vi "0_Augment_Dataset.vi"() -> ()   [LabVIEW 2020]
uses:
  <vilib>/vision/NI_Vision_Development_Module.lvlib
panel:
  out "File Data Type":i32(ring)=5 items=["1 bit", "2 bits", "4 bits", "8 bits", "12 bits (unsigned)", "16 bits (unsigned)", "16 bits (signed)", "16 bits (RGB chunky)", "24 bits (RGB chunky)", "24 bits (RGB planar)", "32 bits (unsigned)", "32 bits (signed)", "32 bits (RGB chunky)", "32 bits (float)", "48 bits (Complex 2x24 int)", "64 bits (Complex 2x32 float)", "reserved", "24 bits (HSL)", "48 bits (RGB chunky)", "64 bits (RGB chunky)"]
  out "Image Type":T1=7 items=["Grayscale (U8)", "Grayscale (I16)", "Grayscale (SGL)", "Complex (CSG)", "RGB (U32)", "HSL (U32)", "RGB (U64)", "Grayscale (U16)"]
  out "error out":errorcluster
  in  "error in (no error)":errorcluster
  in  "Image Path":path=path "D:/Ngene/Projects_SVN/LV_DNN_Projects/2022/2022_09_14_Andrzej Czechowski_Comex/2_Dataset/2022_10_04_Initial_Dataset/orig_train_test_aug_FR0"
  out "No of Images":i32=756
  out "Progress":i32=755
  # "Description:\nThis VI increases datset size by a facor of 8 by applyig vertical and horizontal flipping and rotation by 90, 180 and 270 degrees."
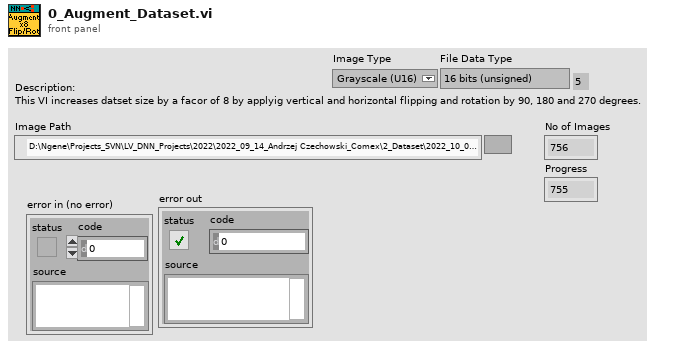
[diagram p1: front panel]
types:
  T1 = typedef "Image Type" = u32
  T2 = typedef "IMAQ Image.ctl" = refnum<image>
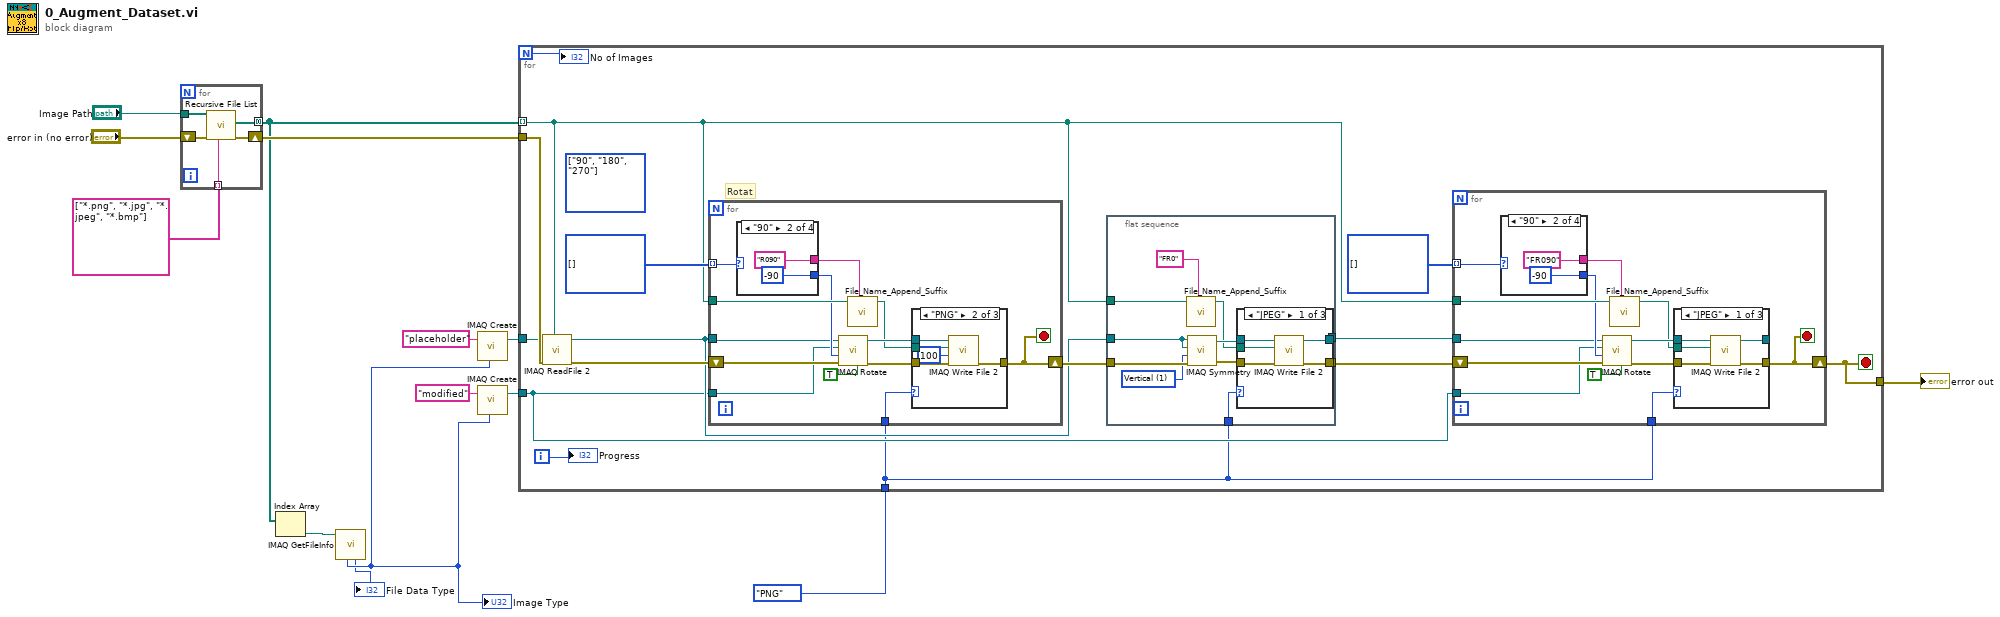
[diagram p0: block diagram]
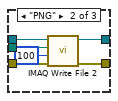
[diagram p2: hidden frame]
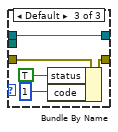
[diagram p3: hidden frame]
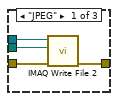
[diagram p4: hidden frame]
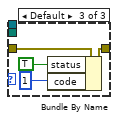
[diagram p5: hidden frame]
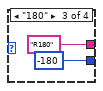
[diagram p7: hidden frame]
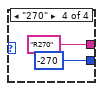
[diagram p8: hidden frame]
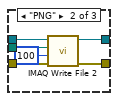
[diagram p9: hidden frame]
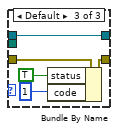
[diagram p10: hidden frame]
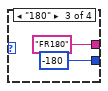
[diagram p12: hidden frame]
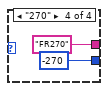
[diagram p13: hidden frame]
diagram:
  n1 = for {
    tunnel: "Image Path" -> [w19]
    tunnel: string[] ["*.png", "*.jpg", "*.jpeg", "*.bmp"] ("pattern") -> [w18] mode=indexing
    tunnel: [w17] -> w5 mode=concatenating
    shift-right: [w15] -> w6
    shift-left: "error in (no error)" -> [w16]
    n2 = call <vilib>:"Recursive File List.vi"("pattern"=w18, "error in (no error)"=w16, "Folder Path"=w19) -> ("error out"=w15:errorcluster, "All Files in Dir"=w17:path[])  [unwired: 4 in, 3 out]
  }
  n3 = Index Array(array=w5) -> (element=w4:path)  [unwired: 1 in]
  n4 = call "IMAQ GetFileInfo"("File Path"=w4) -> ("File Data Type"=→"File Data Type":i32, "Image Type"=w3:T1)  [unwired: 4 in, 5 out]
  "Image Type" <- w3
  n5 = call "IMAQ Create"("Image Name"="placeholder", "Image Type"=w3) -> ("New Image"=w10:T2)  [unwired: 3 in, 1 out]
  n6 = call "IMAQ Create"("Image Name"="modified", "Image Type"=w3) -> ("New Image"=w9:T2)  [unwired: 3 in, 1 out]
  n7 = for {
    N -> [w33]
    tunnel: w5 -> [w22] mode=indexing
    tunnel: w10 -> [w32]
    tunnel: w9 -> [w25]
    tunnel: [w21] -> w7
    tunnel: w6 -> [w34]
    tunnel: enum16{"JPEG", "PNG", "BMP"}."PNG" -> [w20]
    i -> [w23]
    stop <- w21 stop-if-true
    (unwired) enum16{"0", "90", "180", "270"}[] [enum."90", enum."180", enum."270"] items=["0", "90", "180", "270"]
    w26 = enum16{"0", "90", "180", "270"}[] [] items=["0", "90", "180", "270"]
    w31 = enum16{"0", "90", "180", "270"}[] [] items=["0", "90", "180", "270"]
    # "Rotat"
    n8 = call "IMAQ ReadFile 2"("File Path"=w22, "error in (no error)"=w34, "Image"=w32) -> ("error out"=w30:errorcluster, "Image Out"=w28:T2)  [unwired: 4 in, 3 out]
    n9 = for {
      tunnel: w31 -> [w72] mode=indexing
      tunnel: w28 -> [w64]
      tunnel: w22 -> [w71]
      shift-right: [w65] -> w29
      shift-left: w30 -> [w69]
      tunnel: w25 -> [w63]
      tunnel: w20 -> [w62]
      stop <- w65 stop-if-true
      n10 = case shown="\"90\"" w72 {
        tunnel: [_ "R090" "R180" "R270"] -> w67
        tunnel: [_ -90 -180 -270] -> w66
        frame "0", Default {
        }
        frame "90" {
        }
        frame "180" {
        }
        frame "270" {
        }
      }
      n11 = call "IMAQ Rotate"("Use Bilinear Interpolation"=TRUE, "error in (no error)"=w69, "Angle (degrees)"=w66, "Image Dst"=w63, "Image Src"=w64) -> ("error out"=w68:errorcluster, "Image Dst Out"=w73:T2)  [unwired: 5 in]
      n12 = call "File_Name_Append_Suffix.vi"("Suffix"=w67, "Path"=w71) -> ("appended path"=w70:path)  [unwired: 9 in]
      n13 = case shown="\"PNG\"" w62 {
        tunnel: w73 -> [w78 w83 _]
        tunnel: w70 -> [w77 w82 _]
        tunnel: w68 -> [w76 w81 w87]
        tunnel: [w75 w80 w86] -> w65
        frame "JPEG" {
          n14 = call-poly "IMAQ Write File 2"("error in (no error)"=w76, "File Path"=w77, "Image"=w78) -> ("error out"=w75:errorcluster)  [unwired: 7 in, 1 out]
        }
        frame "PNG" {
          n15 = call-poly "IMAQ Write File 2"("error in (no error)"=w81, "Image Quality"=u32 100, "File Path"=w82, "Image"=w83) -> ("error out"=w80:errorcluster)  [unwired: 6 in, 1 out]
        }
        frame Default {
          n16 = Bundle By Name(cluster=w87, "status"=TRUE, "code"=1) -> (w86:errorcluster)
        }
      }
    }
    n17 = flat-sequence {
      tunnel: w28 -> [w42]
      tunnel: w22 -> [w45]
      tunnel: w29 -> [w44]
      tunnel: [w35] -> w27
      tunnel: [w36] -> w24
      tunnel: w20 -> [w37]
      frame #0 {
        w41 = u32 1 items=["Horizontal", "Vertical", "Central", "1st Diagonal", "2nd Diagonal"] ("Type of Symmetry")
        n18 = call "File_Name_Append_Suffix.vi"("Suffix"="FR0", "Path"=w45) -> ("appended path"=w38:path)  [unwired: 9 in]
        n19 = call "IMAQ Symmetry"("error in (no error)"=w44, "Type of Symmetry"=w41, "Image Dst"=w42, "Image Src"=w42) -> ("error out"=w39:errorcluster, "Image Dst Out"=w40:T2)  [unwired: 1 in]
        n20 = case shown="\"JPEG\"" w37 {
          tunnel: w40 -> [w50 w56 w57]
          tunnel: w38 -> [w49 w55 _]
          tunnel: w39 -> [w48 w54 w61]
          tunnel: [w47 w53 w60] -> w35
          tunnel: [w46 w51 w57] -> w36
          frame "JPEG" {
            n21 = call-poly "IMAQ Write File 2"("error in (no error)"=w48, "File Path"=w49, "Image"=w50) -> ("error out"=w47:errorcluster, "Image Out (duplicate)"=w46:T2)  [unwired: 7 in]
          }
          frame "PNG" {
            n22 = call-poly "IMAQ Write File 2"("error in (no error)"=w54, "Image Quality"=u32 100, "File Path"=w55, "Image"=w56) -> ("error out"=w53:errorcluster, "Image Out (duplicate)"=w51:T2)  [unwired: 6 in]
          }
          frame Default {
            n23 = Bundle By Name(cluster=w61, "status"=TRUE, "code"=1) -> (w60:errorcluster)
          }
        }
      }
    }
    n24 = for {
      tunnel: w26 -> [w105] mode=indexing
      tunnel: w24 -> [w100]
      tunnel: w22 -> [w104]
      shift-right: [w94] -> w21
      shift-left: w27 -> [w103]
      tunnel: w25 -> [w99]
      tunnel: w20 -> [w97]
      stop <- w94 stop-if-true
      n25 = case shown="\"90\"" w105 {
        tunnel: [_ "FR090" "FR180" "FR270"] -> w102
        tunnel: [_ -90 -180 -270] -> w101
        frame "0", Default {
        }
        frame "90" {
        }
        frame "180" {
        }
        frame "270" {
        }
      }
      n26 = call "IMAQ Rotate"("Use Bilinear Interpolation"=TRUE, "error in (no error)"=w103, "Angle (degrees)"=w101, "Image Dst"=w99, "Image Src"=w100) -> ("error out"=w96:errorcluster, "Image Dst Out"=w98:T2)  [unwired: 5 in]
      n27 = call "File_Name_Append_Suffix.vi"("Suffix"=w102, "Path"=w104) -> ("appended path"=w95:path)  [unwired: 9 in]
      n28 = case shown="\"JPEG\"" w97 {
        tunnel: w98 -> [w111 w117 w118]
        tunnel: w95 -> [w110 w116 _]
        tunnel: w96 -> [w109 w115 w122]
        tunnel: [w108 w114 w121] -> w94
        tunnel: [w107 w112 w118] -> _
        frame "JPEG" {
          n29 = call-poly "IMAQ Write File 2"("error in (no error)"=w109, "File Path"=w110, "Image"=w111) -> ("error out"=w108:errorcluster, "Image Out (duplicate)"=w107:T2)  [unwired: 7 in]
        }
        frame "PNG" {
          n30 = call-poly "IMAQ Write File 2"("error in (no error)"=w115, "Image Quality"=u32 100, "File Path"=w116, "Image"=w117) -> ("error out"=w114:errorcluster, "Image Out (duplicate)"=w112:T2)  [unwired: 6 in]
        }
        frame Default {
          n31 = Bundle By Name(cluster=w122, "status"=TRUE, "code"=1) -> (w121:errorcluster)
        }
      }
    }
    "No of Images" <- w33
    "Progress" <- w23
  }
  "error out" <- w7
